vi "设控值写入.vi"(0 "表格":string[][](array[string]), 5 "控件配置文件":string[][](array[string]), 7 "DataInitDef":T1 items=["刷新间隔", "波特率", "布尔1设置项", "布尔2设置项", "布尔3设置项", "布尔4设置项", "布尔5设置项", "布尔6设置项", "布尔7设置项", "布尔8设置项", "显控1设置", "显控2设置", "显控3设置", "显控4设置", "显控5设置", "显控6设置", "显控7设置", "显控8设置", "显控9设置", "显控10设置", "显控11设置", "显控12设置", "设控1设置", "设控2设置", "设控3设置", "设控4设置", "设控5设置", "设控6设置", "设控7设置", "设控8设置", "曲线1设置", "曲线2设置", "曲线3设置", "曲线4设置", "曲线5设置", "曲线6设置", "曲线7设置", "曲线8设置", "曲线9设置", "曲线10设置", "曲线11设置", "曲线12设置", "曲线13设置", "曲线14设置", "曲线15设置", "曲线16设置", "曲线17设置", "曲线18设置", "曲线19设置", "曲线20设置", "曲线21设置", "曲线22设置", "曲线23设置", "曲线24设置", "曲线25设置", "曲线26设置", "曲线27设置", "曲线28设置", "曲线29设置", "曲线30设置", "曲线31设置", "曲线32设置", "曲线33设置", "曲线34设置", "曲线35设置", "曲线36设置", "曲线37设置", "曲线38设置", "曲线39设置", "曲线40设置", "曲线41设置", "曲线42设置", "曲线43设置", "曲线44设置", "曲线45设置", "曲线46设置", "曲线47设置", "曲线48设置", "曲线49设置", "曲线50设置", "曲线51设置", "曲线52设置", "曲线53设置", "曲线54设置", "曲线55设置", "曲线56设置", "曲线57设置", "曲线58设置", "曲线59设置", "曲线60设置", "曲线61设置", "曲线62设置", "曲线63设置", "曲线64设置", "ID值", "数据模式"], 9 "NewVal":string, 11 "布尔":bool) -> (4 "输出簇":cluster{u16, i32, i32, i32})   [LabVIEW 2021]
uses:
  controls/DataInitDef.ctl
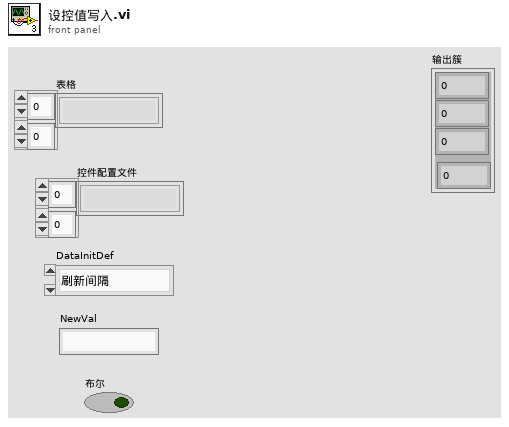
[diagram p1: front panel]
types:
  T1 = typedef "DataInitDef.ctl" = u16
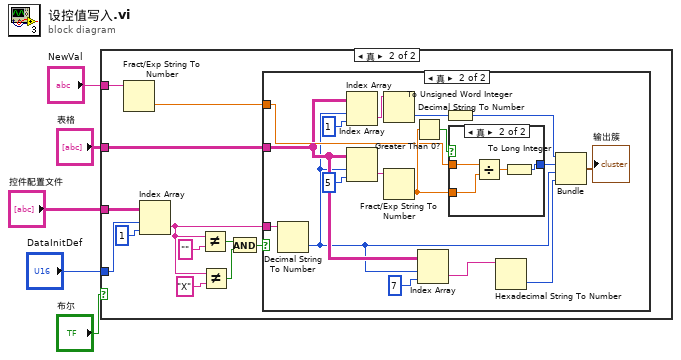
[diagram p0: block diagram]
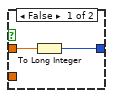
[diagram p4: hidden frame]
diagram:
  n1 = case shown="真" "布尔" {
    tunnel: "NewVal" -> [_ w9]
    tunnel: "控件配置文件" -> [_ w8]
    tunnel: "DataInitDef" -> [_ w7]
    tunnel: "表格" -> [_ w6]
    frame False {
    }
    frame True {
      n2 = Fract/Exp String To Number(string=w9) -> (number=w10:dbl)  [unwired: 3 in, 1 out]
      n3 = Index Array(array=w8, index (row)=w7, index (col)=1 ("禁用的索引 (列)")) -> (element=w15:string)
      n4 = Not Equal?(x=w15, y="") -> (x != y?=w12:bool)
      n5 = Not Equal?(x=w15, y="X") -> (x != y?=w11:bool)
      n6 = And(x=w12, y=w11) -> (x .and. y?=w13:bool)
      n7 = case shown="真" w13 {
        tunnel: w15 -> [_ w33]
        tunnel: w10 -> [_ w25]
        tunnel: w6 -> [_ w20]
        frame False {
        }
        frame True {
          n8 = Decimal String To Number(string=w33) -> (number=w19:i32)  [unwired: 2 in, 1 out]
          n9 = Index Array(array=w20, index (row)=w19, index (col)=1 ("禁用的索引 (列)")) -> (element=w32:string)
          n10 = Index Array(array=w20, index (row)=w19, index (col)=5 ("禁用的索引 (列)")) -> (element=w28:string)
          n11 = Decimal String To Number(string=w32) -> (number=w30:i32)  [unwired: 2 in, 1 out]
          n12 = Fract/Exp String To Number(string=w28) -> (number=w26:dbl)  [unwired: 3 in, 1 out]
          n13 = Greater Than 0?(x=w26) -> (x > 0?=w27:bool)
          n14 = Index Array(array=w20, index (row)=w19, index (col)=7 ("禁用的索引 (列)")) -> (element=w21:string)
          n15 = To Unsigned Word Integer(number=w30) -> (unsigned 16bit integer=w34:u16)
          n16 = case shown="真" w27 {
            tunnel: w26 -> [_ w39]
            tunnel: w25 -> [w36 w38]
            tunnel: [w35 w37] -> w24
            frame False {
              n17 = To Long Integer(number=w36) -> (32bit integer=w35:i32)
            }
            frame True {
              n18 = Divide(x=w38, y=w39) -> (x/y=w40:dbl)
              n19 = To Long Integer(number=w40) -> (32bit integer=w37:i32)
            }
          }
          n20 = Hexadecimal String To Number(string=w21) -> (number=w18:u32)  [unwired: 2 in, 1 out]
          n21 = Bundle(w34, w24, w19, w18) -> (→"输出簇":cluster{u16, i32, i32, u32})  [unwired: 1 in]
        }
      }
    }
  }
